vi "KSD.vi"(0 "System no.":i32=1 min=1 max=4 step=1, 1 "Name":string, 2 "Axes to set":string[](array[string]), 3 "Position values":dbl[](array[numeric]) format="%.6f", 4 "No.of digits":i16=4, 5 "error in":errorcluster) -> (19 "error out":errorcluster)   [LabVIEW 2020]
doc: "Defines a new KSD-type coordinate system in order to set a \"directed\" swivel with the parameters X, Y, Z (relative to the hexapod platform) and queries ERR?. The coordinate system is rotated with the parameters U, V, W. \nIf there is already a coordinate system with the same name, KSD will replace it if it is not used. Activating a KSD type coordinate system (KEN.vi) does not cause any motion, and POS?.vi will report new position values. If the hexapod is moving, the command can be applied. All pivot point coordinates (SPI.vi) will be reset to the previous values after disabling. SPI.vi is not allowed when a KSD type coordinate system is active. For new or replaced KSD type coordinate systems, the parent coordinate system will be set to \"ZERO\". When replacing a coordinate system of this type, the chain relations will not be changed if the coordinate system to replace is of the same type. For axes which are not given, the position values will be set to 0. Coordinate system settings are volatile but can be saved as power-on default with WPA.vi using the password \"SKS\". This command requires command level 0 or 1.\n\nC-887, F-206, M-8X0: Only for GCS syntax version = GCS 2.0 or higher (Check with CSV?.vi. If CSV?.vi is not supported, syntax version is GCS 1.0)."
panel:
  # "Defines a new KSD-type coordinate system in order to set a \"directed\" \nswivel with the parameters X, Y, Z (relative to the Hexapod platform) and\nqueries ERR?. The coordinate system is rotated with the parameters \nU, V, W."
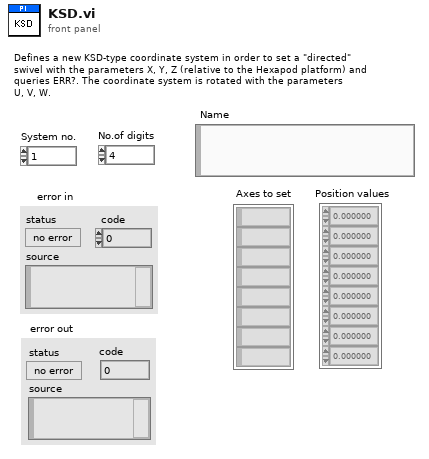
[diagram p1: front panel]
types:
  T1 = enum16{"Disable error check", "Force error check", "Use global settings"}
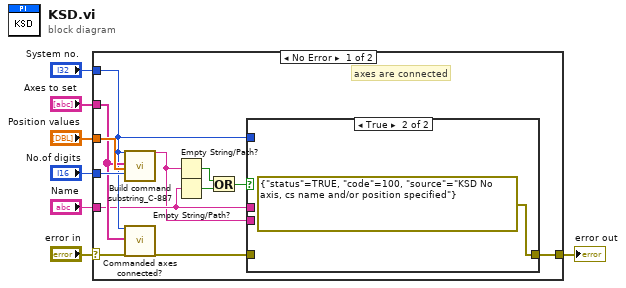
[diagram p0: block diagram]
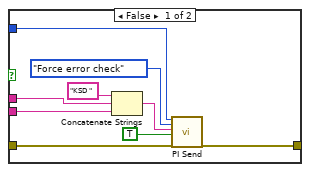
[diagram p2: hidden frame]
diagram:
  n1 = case shown="No Error" "error in" {
    selector: "error in" -> [w12 w30]
    tunnel: [w19 w30] -> w7
    tunnel: "Position values" -> [w18 _]
    tunnel: "No.of digits" -> [w17 _]
    tunnel: "System no." -> [w14 _]
    tunnel: "Axes to set" -> [w15 _]
    tunnel: "Name" -> [w11 _]
    frame No Error {
      # "axes are connected"
      n2 = call "Build command substring_C-887.vi"("System no."=w14, "Affected axes"=w15, "Parameters"=w18, "No. of digits"=w17) -> ("Command substring"=w9:string)  [unwired: 3 in, 12 out]
      n3 = call "Commanded axes connected?.vi"("System no."=w14, "Commanded axes"=w15, "error in"=w12) -> ("error out"=w16:errorcluster)  [unwired: 1 in, 15 out]
      n4 = Empty String/Path?(string/path=w9) -> (empty?=w8:bool)
      n5 = Empty String/Path?(string/path=w11) -> (empty?=w10:bool)
      n6 = Or(x=w8, y=w10) -> (x .or. y?=w13:bool)
      n7 = case shown="True" w13 {
        tunnel: [w21 errorcluster {"status"=TRUE, "code"=100, "source"="KSD No axis, cs name and/or position specified"} ("error out")] -> w19
        tunnel: w9 -> [w28 _]
        tunnel: w16 -> [w27 _]
        tunnel: w14 -> [w22 _]
        tunnel: w11 -> [w26 _]
        frame False {
          n8 = Concatenate Strings("KSD ", w26, w28) -> (w24:string)
          n9 = call "PI Send.vi"("System no."=w22, "Error check settings"=T1."Force error check", "String to send"=w24, "Attach termination char.?"=TRUE ("Attach Linefeed?"), "error in"=w27) -> ("error out"=w21:errorcluster)  [unwired: 1 in, 13 out]
        }
        frame True {
        }
      }
    }
    frame Error {
    }
  }
  "error out" <- w7
